vi "GetSNR(SubVI).vi"(9 "noise length from tail (50)":i32=50, 11 "Waveform":dbl[](array[numeric])) -> (3 "SNR":dbl)   [LabVIEW 2024]
uses:
  <vilib>/Analysis/NI_AALBase.lvlib
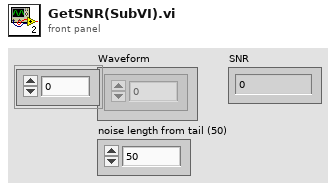
[diagram p1: front panel]
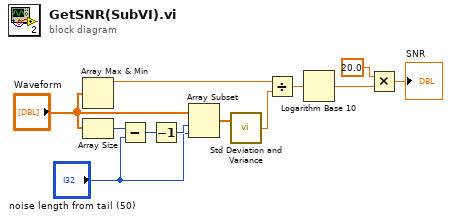
[diagram p0: block diagram]
diagram:
  n1 = Array Max & Min(array="Waveform") -> (max value=w7:dbl)  [unwired: 3 out]
  n2 = Array Size(array="Waveform") -> (size(s)=w2:i32)
  n3 = Subtract(x=w2, y="noise length from tail (50)") -> (x-y=w4:i32)
  n4 = Decrement(x=w4) -> (x-1=w5:i32)
  n5 = Array Subset(array="Waveform", index=w5, length="noise length from tail (50)") -> (w6:dbl[])
  n6 = call <vilib>:"Std Deviation and Variance.vi"("X"=w6) -> ("standard deviation"=w8:dbl)  [unwired: 1 in, 2 out]
  n7 = Divide(x=w7, y=w8) -> (x/y=w9:dbl)
  n8 = Logarithm Base 10(1:w9) -> (0:w11:dbl)
  n9 = Multiply(x=20.0, y=w11) -> (x*y=→"SNR":dbl)
